vi "ServerTestVI.vi"() -> ()   [LabVIEW 2018]
uses:
  TCP_Server/TCP_Server.lvclass
panel:
  in  "stop":bool
  out "error out":errorcluster
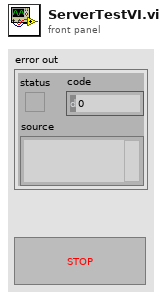
[diagram p1: front panel]
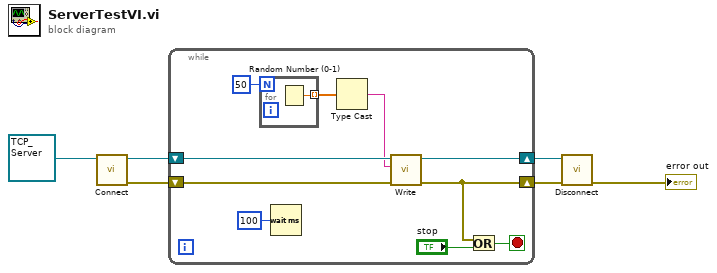
[diagram p0: block diagram]
diagram:
  n1 = call-dynamic "Connect.vi"("TCP_Server in"=refnum<class "TCP_Server.lvclass"> refnum ("TCP_Server.lvlib:TCP_Server.lvclass")) -> ("error out"=w5:errorcluster, "TCP_Server out"=w6:refnum<class "TCP_Server.lvclass">)  [unwired: 9 in]
  n2 = while {
    shift-right: [w14] -> w4
    shift-left: w6 -> [w16]
    shift-right: [w13] -> w3
    shift-left: w5 -> [w15]
    stop <- w11 stop-if-true
    n3 = for {
      N: 50 ("# of Points") -> [_]
      tunnel: [w17] -> w8 mode=indexing
      n4 = Random Number (0-1)() -> (number: 0 to 1=w17:dbl)
    }
    n5 = Wait (ms)(milliseconds to wait=u32 100) -> ()  [unwired: 1 out]
    n6 = Type Cast(x=w8) -> (*(type *) &x=w7:string)  [unwired: 1 out]
    n7 = call-dynamic "Write.vi"("error in (no error)"=w15, "Message"=w7, "TCP_Client in"=w16) -> ("error out"=w13:errorcluster, "TCP_Client out"=w14:refnum<class "TCP_Server.lvclass">)  [unwired: 7 in]
    n8 = Or(x=w13, y="stop") -> (x .or. y?=w11:bool)
  }
  n9 = call-dynamic "Disconnect.vi"("error in (no error)"=w3, "TCP_Client in"=w4) -> ("error out"=→"error out":errorcluster)  [unwired: 8 in, 1 out]
